vi "FTP_DecodeDirString.vi"(6 "directory":string, 7 "name":string) -> (0 "before substring":string, 1 "file elements":string[](array[string]), 2 "On Server?":bool, 3 "New Format?":bool, 4 "Folder name":string)   [LabVIEW 2012]
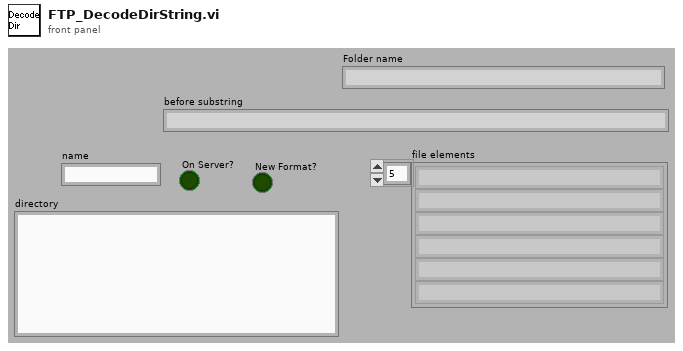
[diagram p1: front panel]
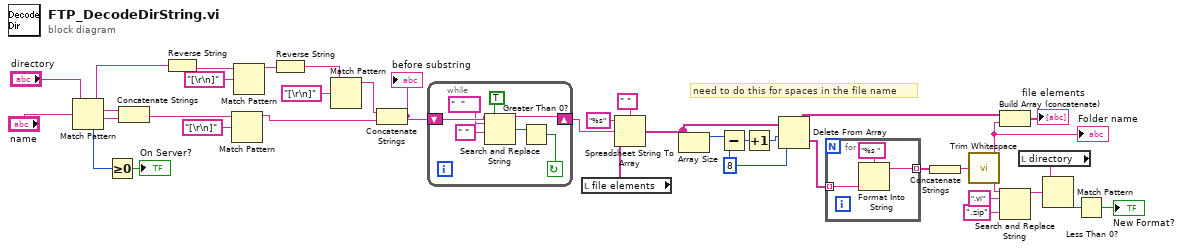
[diagram p0: block diagram]
diagram:
  w15 = 8 ("index")
  # "need to do this for spaces in the file name"
  n1 = Match Pattern(string="directory", regular expression="name") -> (before substring=w22:string, match substring=w33:string, after substring=w34:string, offset past match=w21:i32)  [unwired: 1 out]
  n2 = Greater Or Equal To 0?(x=w21) -> (x >= 0?=→"On Server?":bool)
  n3 = Concatenate Strings(w33, w34) -> (w35:string)
  n4 = Reverse String(1:w22) -> (0:w24:string)
  n5 = Match Pattern(string=w35, regular expression="[\r\n]") -> (before substring=w36:string)  [unwired: 4 out]
  n6 = Match Pattern(string=w24, regular expression="[\r\n]") -> (before substring=w25:string)  [unwired: 4 out]
  n7 = Reverse String(1:w25) -> (0:w27:string)
  n8 = Match Pattern(string=w27, regular expression="[\r\n]") -> (before substring=w37:string)  [unwired: 4 out]
  n9 = Concatenate Strings(w37, w36) -> (w38:string)
  "before substring" <- w38
  n10 = while {
    shift-right: [w41] -> w30
    shift-left: w38 -> [w44]
    stop <- w45 continue-if-true
    n11 = Search and Replace String(replace all?=TRUE ("replace all? (F)"), input string=w44, search string="  ", replace string=" " ("replace string (\"\")")) -> (result string=w41:string, number of replacements=w39:i32)  [unwired: 1 in, 5 out]
    n12 = Greater Than 0?(x=w39) -> (x > 0?=w45:bool)
  }
  n13 = local read "file elements"() -> (w18:string[])
  n14 = Spreadsheet String To Array(delimiter (Tab)=" ", format string="%s", spreadsheet string=w30, array type (2D Dbl)=w18) -> (array=w17:string[])
  n15 = Array Size(array=w17) -> (size(s)=w16:i32)
  n16 = Subtract(x=w16, y=w15) -> (x-y=w14:i32)
  n17 = Increment(x=w14) -> (x+1=w13:i32)
  n18 = Delete From Array(array=w17, length=w13, index=w15) -> (deleted portion=w10:string[], array with subset deleted=w12:string[])
  n19 = for {
    tunnel: w10 -> [w48] mode=indexing
    tunnel: [w47] -> w9 mode=indexing
    n20 = Format Into String(format string="%s ", w48) -> (resulting string=w47:string)  [unwired: 2 in, 1 out]
  }
  n21 = Concatenate Strings(w9) -> (w8:string)
  n22 = call <vilib>:"Trim Whitespace.vi"("string"=w8) -> ("trimmed string"=w7:string)  [unwired: 1 in]
  "Folder name" <- w7
  n23 = Build Array (concatenate)(w12, w7) -> (→"file elements":string[])
  n24 = Search and Replace String(input string=w7, search string=".vi", replace string=".zip" ("replace string (\"\")")) -> (result string=w3:string)  [unwired: 1 in, 7 out]
  n25 = local read "directory"() -> (w4:string)
  n26 = Match Pattern(string=w4, regular expression=w3) -> (offset past match=w2:i32)  [unwired: 4 out]
  n27 = Less Than 0?(x=w2) -> (x < 0?=→"New Format?":bool)
